vi "11. save waveforms simple.vi"() -> ()   [LabVIEW 2018]
uses:
  <vilib>/MakerHub/LINX/Public/Utilities/Open Serial.vi
  <vilib>/Waveform/WDTFileIO.llb/ Write Waveforms to File (1D).vi
  <vilib>/MakerHub/LINX/LMH-LINX.lvlib
panel:
  in  "VISA resource":refnum<visa-resource-name>
  in  "Save Waveform?":bool
  in  "stop":bool
  out "Saved Waveforms":waveform(dbl)[](graph)
  in  "Sampling duration (sec)":dbl=600.0
  in  "Acquition Speed":dbl=200.0
  in  "Analog Input Pin":u8
  out "Normalized Waveform":waveform(dbl)(graph)
  out "Waveform":waveform(dbl)(graph)
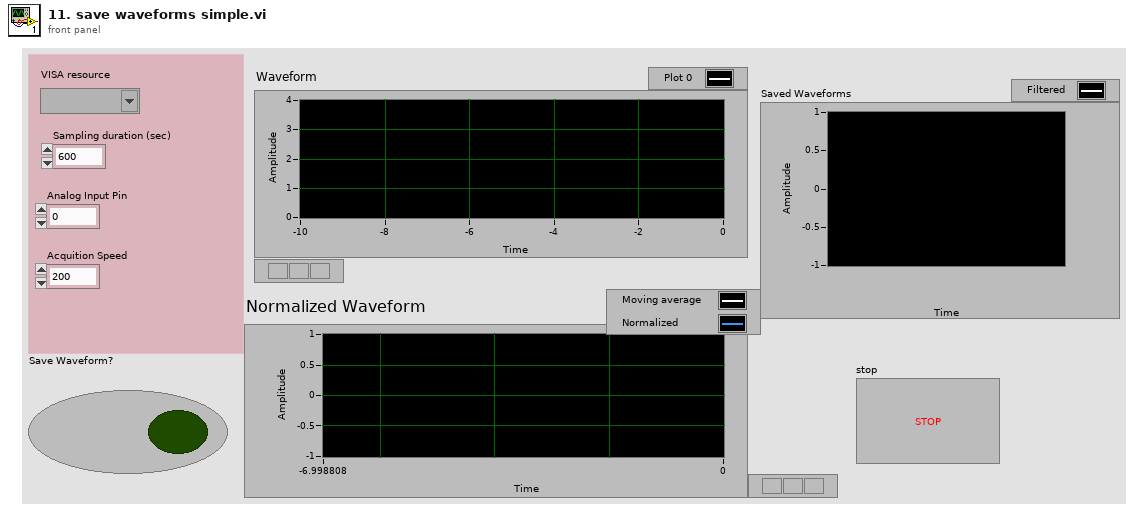
[diagram p1: front panel]
types:
  T1 = typedef "LMH-LINX.lvlib/LINX Ref.ctl" = cluster{"IO":T2, "Interface":T3, "LINX Device Config":T4}
  T2 = typedef "LMH-LINX.lvlib/Platform.ctl" = enum16{"Remote", "Local"}
  T3 = typedef "LMH-LINX.lvlib/Interface.ctl" = enum16{"Serial", "TCP"}
  T4 = typedef "LMH-LINX.lvlib/Device.lvlib/LINX Device Config.ctl" = cluster{"Interface":T3, "COM Port":refnum<visa-resource-name>, "TCP Configuration":T5, "Device Family":u8, "Device ID":u8, "Device Name":string, "TCP Ref":refnum<k5>, "Channels":T6}
  T5 = typedef "LMH-LINX.lvlib/Device.lvlib/TCP Config.ctl" = cluster{"IP Address":string, "Port":u16}
  T6 = typedef "LMH-LINX.lvlib/Channels.ctl" = cluster{"DI":u8[], "DO":u8[], "AI":u8[], "AO":u8[], "PWM":u8[], "QE":u8[], "UART":u8[], "I2C 2":u8[], "SPI":u8[], "CAN":u8[], "Servo":u8[], "AI Ref (V)":dbl, "AI Resolution (Bits)":u8, "AO Ref (V)":dbl, "AO Resolution (Bits)":u8}
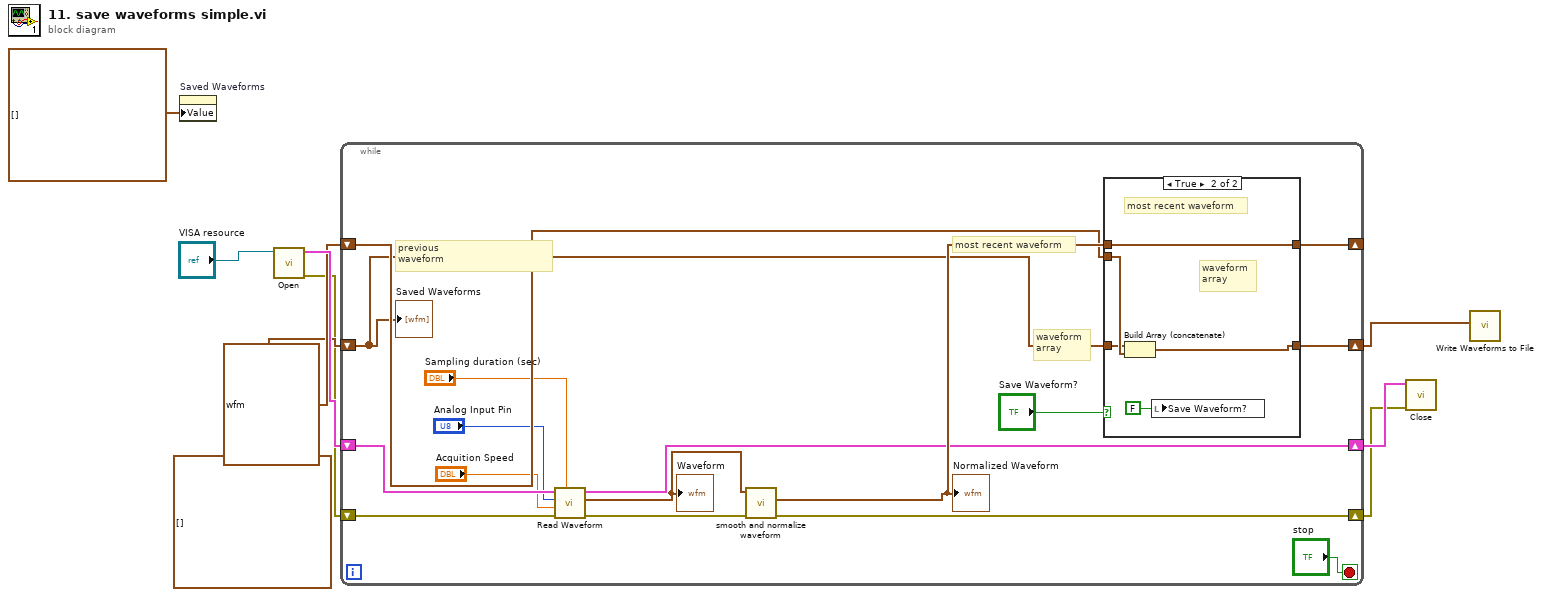
[diagram p0: block diagram]
diagram:
  n1 = property on="Saved Waveforms" class="WFChart (strict)"("Value"=waveform(dbl)[] [] ("Saved Waveforms")) -> ()  [unwired: 2 in, 2 out]
  n2 = call-poly <vilib>:"Open.vi"("Serial Port"="VISA resource") -> ("Error Out"=w3:errorcluster, "LINX Resource"=w9:T1)  [unwired: 8 in, 1 out]
  n3 = while {
    shift-right: [w20] -> _
    shift-left: waveform(dbl) {"t0"=timestamp(0 s since 1904-01-01), "dt"=1.0, "Y"=[]} ("Waveform") -> [w22]
    shift-right: [w21] -> w8
    shift-left: waveform(dbl)[] [] -> [w19]
    shift-right: [w11] -> w2
    shift-left: w9 -> [w25]
    shift-right: [w10] -> w1
    shift-left: w3 -> [w18]
    stop <- "stop" stop-if-true
    # "most recent waveform"
    # "previous\nwaveform"
    # "waveform\narray"
    n4 = call "Read Waveform.vi"("Sampling duration (s)"="Sampling duration (sec)", "error in (no error)"=w18, "Sampling freq (Hz)"="Acquition Speed", "Analog Channel"="Analog Input Pin", "LINX Resource in"=w25) -> ("error out"=w13:errorcluster, "Waveform out"=w14:waveform(dbl), "LINX Resource out"=w11:T1)  [unwired: 1 in, 1 out]
    "Waveform" <- w14
    n5 = call "smooth and normalize waveform.vi"("error in (no error)"=w13, "waveform in"=w14) -> ("error out"=w10:errorcluster, "smoothed and normalized  waveform"=w23:waveform(dbl))  [unwired: 7 in, 1 out]
    "Normalized Waveform" <- w23
    n6 = case shown="True" "Save Waveform?" {
      tunnel: [w27 w32] -> w20
      tunnel: w23 -> [w27 w32]
      tunnel: [w26 w31] -> w21
      tunnel: w22 -> [_ w29]
      tunnel: w19 -> [w26 w28]
      frame False {
        # "most recent waveform"
      }
      frame True {
        # "waveform\narray"
        # "most recent waveform"
        n7 = Build Array (concatenate)(w28, w29) -> (w31:waveform(dbl)[])
        n8 = local write "Save Waveform?"(FALSE ("Save Waveform?")) -> ()
      }
    }
    "Saved Waveforms" <- w19
  }
  n9 = call <vilib>:"Close.vi"("Error In"=w1, "LINX Resource"=w2) -> ()  [unwired: 9 in, 1 out]
  n10 = call-poly <vilib>:"Write Waveforms to File.vi"("waveform array"=w8) -> ()  [unwired: 9 in, 2 out]
